vi "Host.vi"() -> ()   [LabVIEW 2018]
uses:
  <instrlib>/niDCPower/nidcpower.llb/niDCPower Source Mode.ctl
  REMOTE_SEE_CONTROLLER/RemoteSeeAbleService.dll
  <instrlib>/niDCPower/nidcpower.llb/niDCPower Measurement Type.ctl
panel:
  in  "Wait ExamineSee, ms":u32=10
  in  "Wait CheckSee, ms":u32=10
  in  "TryParrySeeDone":bool
  in  "StartTryParrySee":bool
  in  "ShutdownDone":bool
  in  "StartShutdown":bool
  in  "IsParryable":bool
  in  "ExamineSeeDone":bool
  in  "StartExamineSee":bool
  in  "CheckSeeDone":bool
  in  "StartCheckSee":bool
  in  "SeeInfo":string
  in  "IsIncomplete":bool
  in  "IsSee":bool
  in  "Wait_after, ms":u32=10
  in  "Wait before, ms":u32=10
  in  "Wait on, ms":u32=500
  in  "SEL Reset, ms":u32=500
  in  "Тип файла":enum32{"Excel", "Text"}(radio)
  in  "Стоп":bool
  in  "V1.1":bool caption="Питание"
  in  "V1.0":bool caption="Питание"
  in  "V0.1":bool caption="Питание"
  in  "V0.0":bool caption="Питание"
  out "V1.0 bulb SEL":bool
  out "V0.0 bulb SEL":bool
  in  "Лог":path
  in  "SIM_SEL":bool caption="Имитатор\nтиристора"
  in  "V1.0_selcur":dbl=0.01 caption="Порог тиристора" format="%_6p"
  in  "V0.1_selcur":dbl=0.01 caption="Порог тиристора" format="%_6p"
  in  "V1.1_selcur":dbl=0.01 caption="Порог тиристора" format="%_6p"
  in  "V0.0_selcur":dbl=0.01 caption="Порог тиристора" format="%_6p"
  out "V0.0":u16 caption="Счетчик тиристора"
  out "V1.1":u16 caption="Счетчик тиристора"
  out "V0.1":u16 caption="Счетчик тиристора"
  out "V1.0":u16 caption="Счетчик тиристора"
  out "V1.1 bulb SEL":bool
  out "V0.1 bulb SEL":bool
  in  "Питание":bool caption="Общее питание"
  in  "PXI источник №2":refnum<k15>="PXI1Slot3_3" caption="1"
  in  "PXI источник №1":refnum<k15>="PXI1Slot2_2"
  out "V0.0_char":dbl(graph)=3.090307114174992e-07
  out "V1.1_char":dbl(graph)=7.013574706441118e-05
  in  "V0.0":dbl=1.8 caption="Напряжение" format="%_6p"
  out "V0.0_cur":dbl caption="Ток" format="%_6g"
  out "V1.1_cur":dbl caption="Ток" format="%_6g"
  in  "V0.0_curlim":dbl=0.015 caption="Предел тока" format="%_6p"
  in  "V1.1_curlim":dbl=0.015 caption="Предел тока" format="%_6p"
  in  "V1.1":dbl=1.8 caption="Напряжение" format="%_6p"
  out "V0.1_char":dbl(graph)=1.1897542296492405e-06
  out "V1.0_char":dbl(graph)=9.386918666795367e-05
  in  "V0.1":dbl=1.8 caption="Напряжение" format="%_6p"
  out "V0.1_cur":dbl caption="Ток" format="%_6g"
  out "V1.0_cur":dbl caption="Ток" format="%_6g"
  in  "V0.1_curlim":dbl=0.015 caption="Предел тока" format="%_6p"
  in  "V1.0_curlim":dbl=0.015 caption="Предел тока" format="%_6p"
  in  "V1.0":dbl=1.8 caption="Напряжение" format="%_6p"
  # "Канал 1"
  # "Канал 1"
  # "Канал 2"
  # "Канал 2"
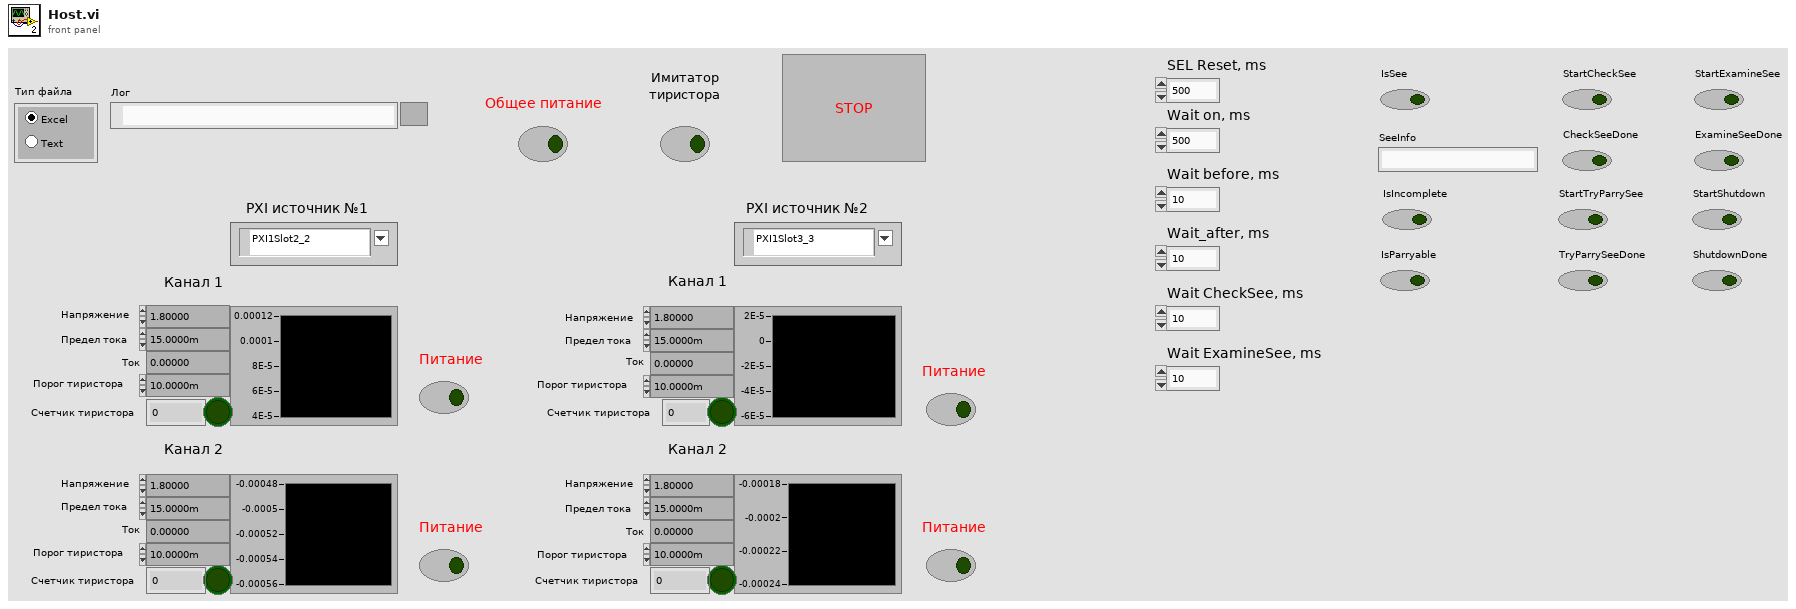
[diagram p1: front panel]
types:
  T1 = enum16{"open", "replace", "create", "open or create", "replace or create", "replace or create with confirmation"}
  T2 = typedef "niDCPower Source Mode.ctl" = i32
  T3 = cluster{"StartCheckSee":refnum<vi>, "CheckSeeDone":refnum<vi>, "IsSee":refnum<vi>, "SeeInfo":refnum<vi>, "IsIncomplete":refnum<vi>}
  T4 = cluster{"StartExamineSee":refnum<vi>, "ExamineSeeDone":refnum<vi>, "IsSee":refnum<vi>, "SeeInfo":refnum<vi>, "IsIncomplete":refnum<vi>}
  T5 = cluster{"StartShutdown":refnum<vi>, "ShutdownDone":refnum<vi>}
  T6 = cluster{"StartTryParrySee":refnum<vi>, "TryParrySeeDone":refnum<vi>}
  T7 = typedef "niDCPower Measurement Type.ctl" = i32
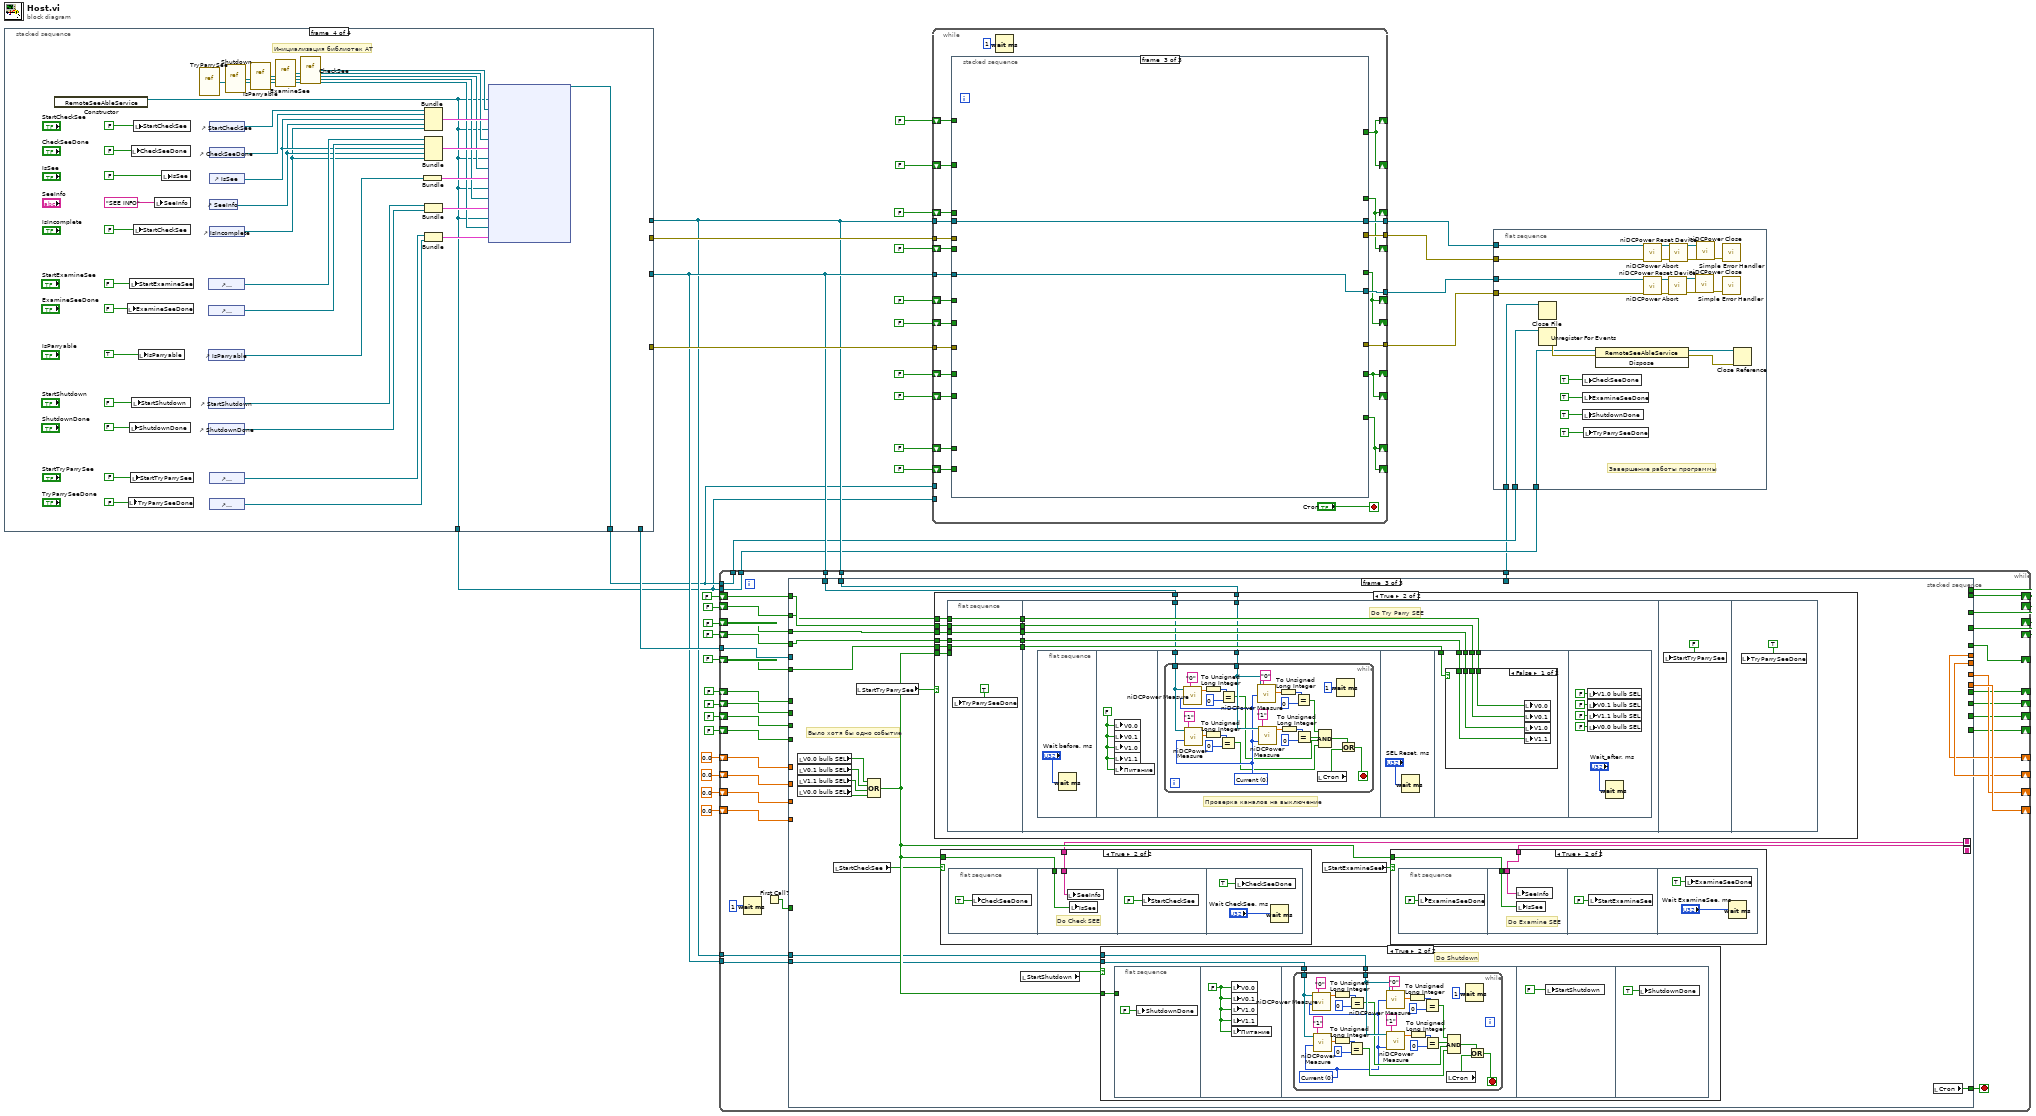
[diagram p0: block diagram]
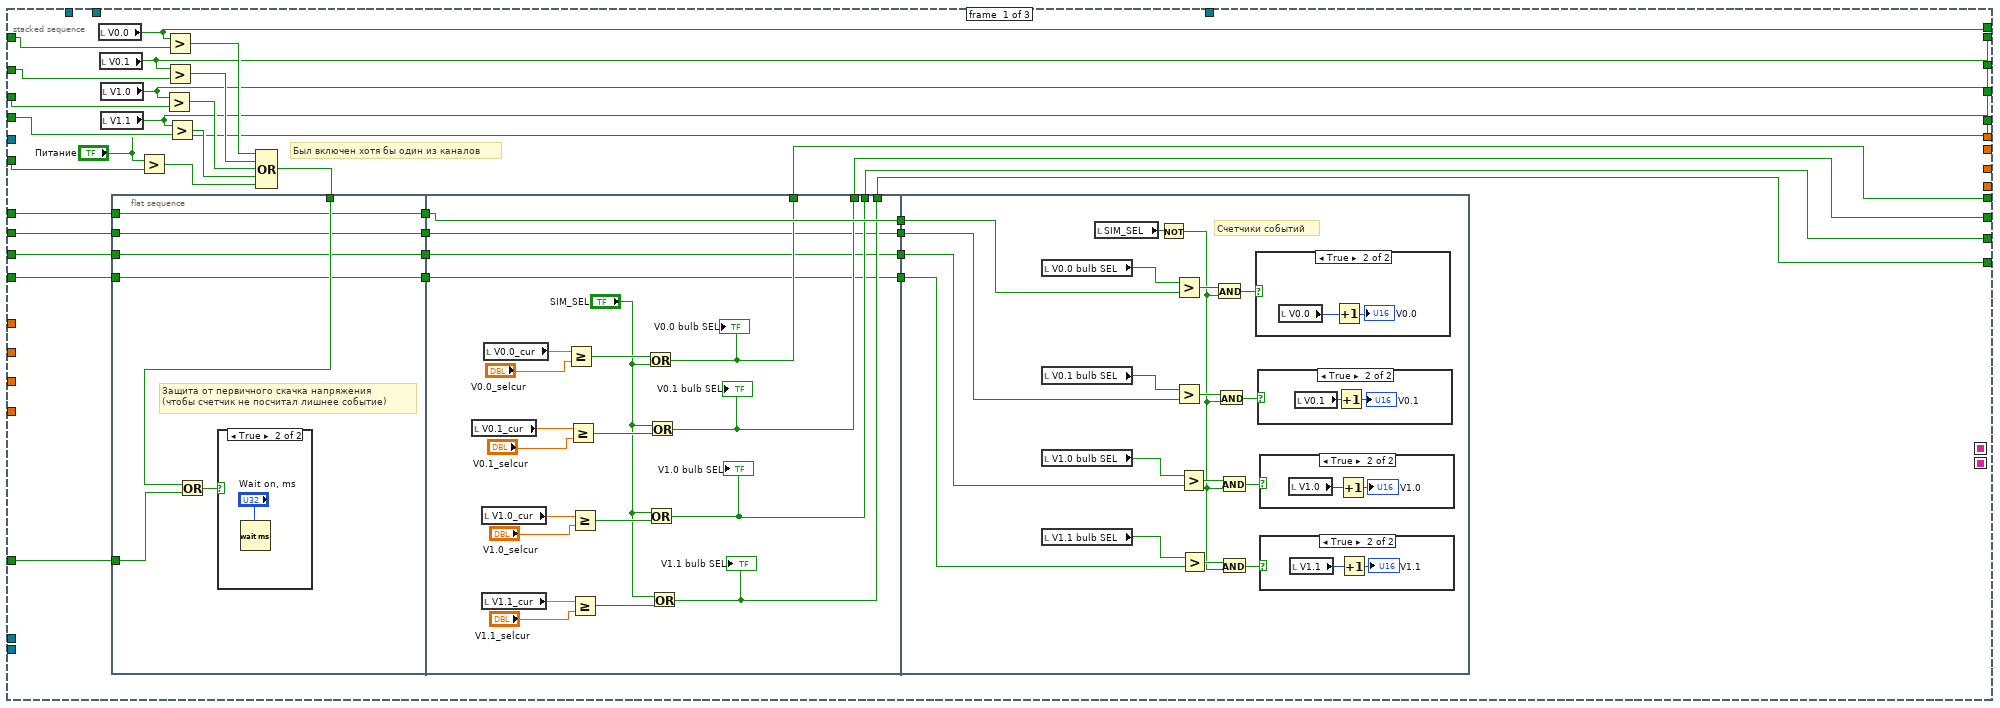
[diagram p2: hidden frame]
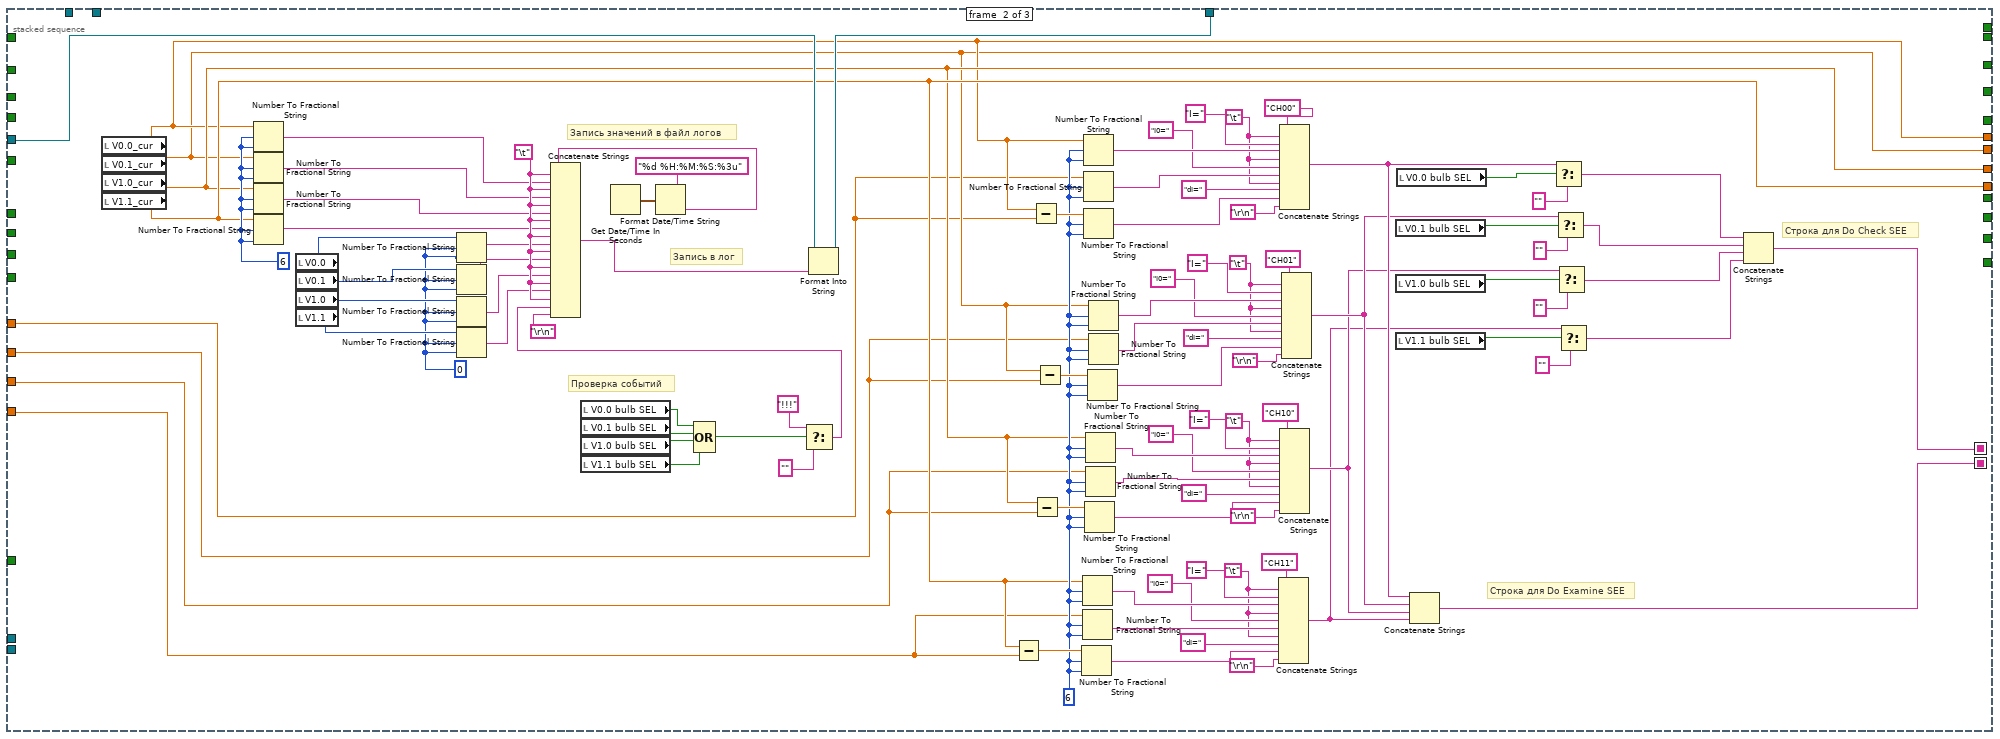
[diagram p8: hidden frame]
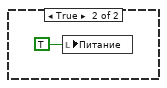
[diagram p10: hidden frame]
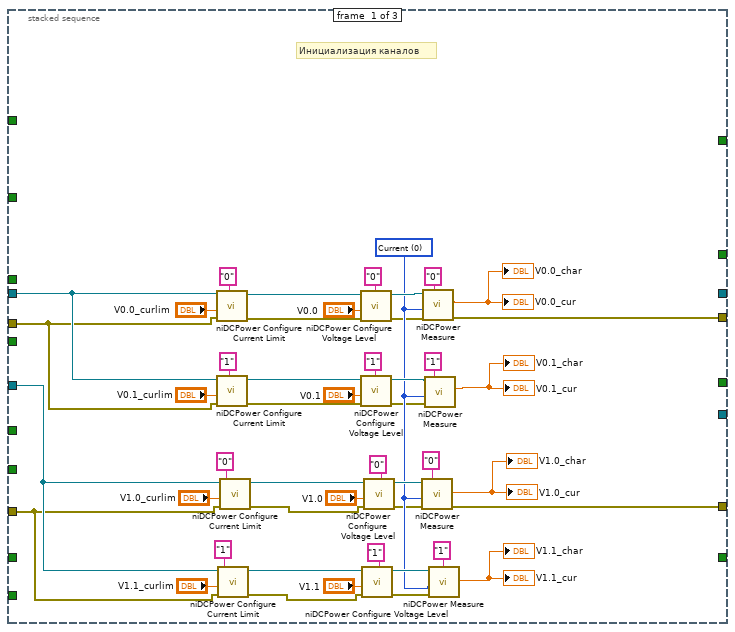
[diagram p14: hidden frame]
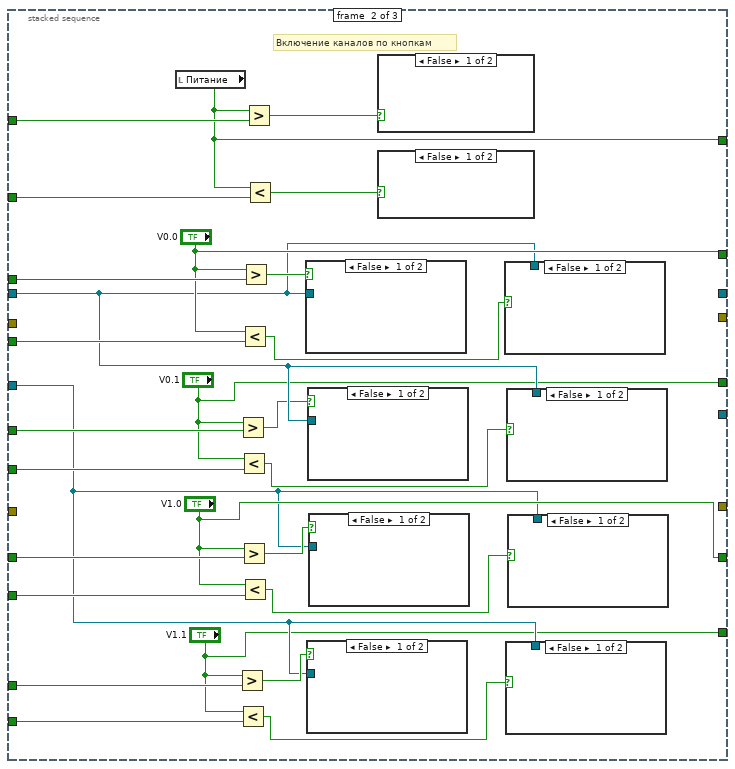
[diagram p15: hidden frame]
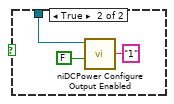
[diagram p16: hidden frame]
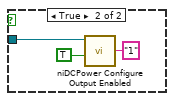
[diagram p17: hidden frame]
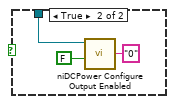
[diagram p18: hidden frame]
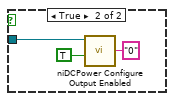
[diagram p19: hidden frame]
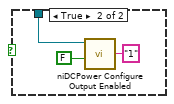
[diagram p20: hidden frame]
diagram:
  n1 = stacked-sequence {
    tunnel: [_ _ w85 _] -> w22
    tunnel: [_ _ w81 _] -> w23
    tunnel: [_ w44 _ _] -> w37
    tunnel: [_ _ w79 _] -> w29
    tunnel: [_ _ w78 _] -> w28
    tunnel: [_ _ _ w101] -> w10
    tunnel: [_ _ _ w102] -> w9
    frame #0 {
      w39 = u16 0
      w38 = FALSE
      # "Начальные значения переменных"
      n2 = local write "V1.0 bulb SEL"(w38) -> ()
      n3 = local write "V1.1 bulb SEL"(w38) -> ()
      n4 = local write "V0.0 bulb SEL"(w38) -> ()
      n5 = local write "V0.1 bulb SEL"(w38) -> ()
      n6 = local write "V0.1 bulb SEL"(w38) -> ()
      n7 = local write "Питание"(w38) -> ()
      n8 = local write "SIM_SEL"(w38) -> ()
      n9 = local write "Стоп"(w38) -> ()
      n10 = local write "V1.0"(w38) -> ()
      n11 = local write "V1.1"(w38) -> ()
      n12 = local write "V0.0"(w38) -> ()
      n13 = local write "V0.1"(w38) -> ()
      n14 = local write "V1.0"(w39) -> ()
      n15 = local write "V0.1"(w39) -> ()
      n16 = local write "V1.1"(w39) -> ()
      n17 = local write "V0.0"(w39) -> ()
    }
    frame #1 {
      w50 = "\t"
      # "Инициализация файла логов"
      n18 = call "Begin.vi"() -> ("Образец № 2"=w46:string)  [unwired: 9 in]
      n19 = Build Path(base path="Лог", name or relative path=w46) -> (appended path=w66:path)
      n20 = Get Date/Time In Seconds() -> (seconds since 1Jan1904=w63:timestamp)
      n21 = call <vilib>:"Check if File or Folder Exists.vi"("path"=w66) -> ("file or folder exists?"=w65:bool, "dup path"=w64:path)  [unwired: 8 in, 1 out]
      n22 = Format Date/Time String(time format string (%c)="%d %H.%M.%S", seconds (now)=w63) -> (date/time string=w62:string)  [unwired: 1 in]
      n23 = case shown="True" w65 {
        tunnel: w64 -> [w72 w73]
        tunnel: [w71 w73] -> w41
        frame False {
          n24 = Create Folder(path (use dialog)=w72) -> (created path=w71:path)  [unwired: 2 in, 2 out]
        }
        frame True {
        }
      }
      n25 = case shown="\"Text\"" "Тип файла" {
        tunnel: [".xls" ("string") ".txt" ("string")] -> w61
        tunnel: w41 -> [w67 w69]
        tunnel: [w67 w69] -> w40
        frame "Excel", Default {
        }
        frame "Text" {
        }
      }
      n26 = Concatenate Strings(w62, w61) -> (w59:string)
      n27 = Build Path(base path=w40, name or relative path=w59) -> (appended path=w56:path)
      n28 = Open/Create/Replace File(file path (use dialog)=w56, operation (0:open)=T1."open or create", access (0:read/write)=enum16{"read/write", "read-only", "write-only"}."read/write") -> (refnum out=w48:refnum<file>)  [unwired: 3 in, 2 out]
      n29 = Set File Position(refnum=w48, from (0:start)=enum16{"start", "end", "current"}."end") -> (refnum out=w45:refnum<file>)  [unwired: 2 in, 1 out]
      n30 = Format Into String(initial string=w45, "Time" ("string"), w50, " V 0.0" ("string"), w50, "V 0.1" ("string"), w50, "V 1.0" ("string"), w50, "V 1.1" ("string"), w50, "\r\n") -> (resulting string=w44:refnum<file>)  [unwired: 2 in, 1 out]
    }
    frame #2 {
      w86 = T2 1020 items=["Single Point"=1020, "Sequence"=1021] ("source mode")
      w92 = T2 1020 items=["Single Point"=1020, "Sequence"=1021] ("source mode")
      # "Инициализация источников"
      n31 = call <instrlib>:"niDCPower Initialize With Channels.vi"("channels"="0,1", "resource name"="PXI источник №1") -> ("error out"=w88:errorcluster, "instrument handle out"=w91:refnum<k15>)  [unwired: 8 in]
      n32 = call <instrlib>:"niDCPower Initialize With Channels.vi"("channels"="0,1", "resource name"="PXI источник №2") -> ("error out"=w93:errorcluster, "instrument handle out"=w95:refnum<k15>)  [unwired: 8 in]
      n33 = call <instrlib>:"niDCPower Configure Source Mode.vi"("error in (no error)"=w93, "source mode"=w92, "instrument handle"=w95) -> ("error out"=w87:errorcluster, "instrument handle out"=w94:refnum<k15>)  [unwired: 7 in]
      n34 = call <instrlib>:"niDCPower Configure Source Mode.vi"("error in (no error)"=w88, "source mode"=w86, "instrument handle"=w91) -> ("error out"=w89:errorcluster, "instrument handle out"=w90:refnum<k15>)  [unwired: 7 in]
      n35 = call <instrlib>:"niDCPower Configure Voltage Level.vi"("error in (no error)"=w87, "voltage level"=0.0, "channel name"="0,1", "instrument handle"=w94) -> ("error out"=w83:errorcluster, "instrument handle out"=w82:refnum<k15>)  [unwired: 6 in]
      n36 = call <instrlib>:"niDCPower Configure Voltage Level.vi"("error in (no error)"=w89, "voltage level"=0.0, "channel name"="0,1", "instrument handle"=w90) -> ("error out"=w80:errorcluster, "instrument handle out"=w84:refnum<k15>)  [unwired: 6 in]
      n37 = call <instrlib>:"niDCPower Initiate.vi"("error in (no error)"=w80, "instrument handle"=w84) -> ("error out"=w79:errorcluster, "instrument handle out"=w85:refnum<k15>)  [unwired: 2 in, 6 out]
      n38 = call <instrlib>:"niDCPower Initiate.vi"("error in (no error)"=w83, "instrument handle"=w82) -> ("error out"=w78:errorcluster, "instrument handle out"=w81:refnum<k15>)  [unwired: 2 in, 6 out]
    }
    frame #3 {
      # "Инициализация библиотек АТ"
      n39 = constructor class="RemoteSeeAbleService"() -> (reference out=w102:refnum<k24>)  [unwired: 3 in, 2 out]
      n40 = local write "ExamineSeeDone"(FALSE ("StartCheckSee")) -> ()
      n41 = local write "TryParrySeeDone"(FALSE ("StartCheckSee")) -> ()
      n42 = local write "StartExamineSee"(FALSE ("StartCheckSee")) -> ()
      n43 = local write "ShutdownDone"(FALSE ("StartCheckSee")) -> ()
      n44 = local write "StartTryParrySee"(FALSE ("StartCheckSee")) -> ()
      n45 = local write "CheckSeeDone"(FALSE ("StartCheckSee")) -> ()
      n46 = local write "StartShutdown"(FALSE ("StartCheckSee")) -> ()
      n47 = local write "StartCheckSee"(FALSE ("StartCheckSee")) -> ()
      n48 = local write "StartCheckSee"(FALSE ("StartCheckSee")) -> ()
      n49 = local write "IsParryable"(TRUE ("StartCheckSee")) -> ()
      n50 = local write "SeeInfo"("SEE INFO" ("SeeInfo")) -> ()
      n51 = local write "IsSee"(FALSE ("StartCheckSee")) -> ()
      n52 = vi-ref "TryParrySee.vi"() -> ("vi reference"=w103:refnum<vi>)
      n53 = control-ref of="StartExamineSee"() -> (w125:refnum<vi>)
      n54 = control-ref of="ExamineSeeDone"() -> (w124:refnum<vi>)
      n55 = control-ref of="IsParryable"() -> (w118:refnum<vi>)
      n56 = control-ref of="StartShutdown"() -> (w114:refnum<vi>)
      n57 = control-ref of="ShutdownDone"() -> (w113:refnum<vi>)
      n58 = control-ref of="StartCheckSee"() -> (w100:refnum<vi>)
      n59 = control-ref of="CheckSeeDone"() -> (w134:refnum<vi>)
      n60 = control-ref of="IsSee"() -> (w123:refnum<vi>)
      n61 = control-ref of="SeeInfo"() -> (w122:refnum<vi>)
      n62 = control-ref of="IsIncomplete"() -> (w121:refnum<vi>)
      n63 = control-ref of="StartTryParrySee"() -> (w109:refnum<vi>)
      n64 = control-ref of="TryParrySeeDone"() -> (w108:refnum<vi>)
      n65 = vi-ref "Shutdown.vi"() -> ("vi reference"=w104:refnum<vi>)
      n66 = vi-ref "IsParryable.vi"() -> ("vi reference"=w105:refnum<vi>)
      n67 = vi-ref "ExamineSee.vi"() -> ("vi reference"=w106:refnum<vi>)
      n68 = vi-ref "CheckSee.vi"() -> ("vi reference"=w133:refnum<vi>)
      n69 = Bundle("IsParryable"=w118) -> (w117:cluster{"IsParryable":refnum<vi>})  [unwired: 1 in]
      n70 = Bundle("StartCheckSee"=w100, "CheckSeeDone"=w134, "IsSee"=w123, "SeeInfo"=w122, "IsIncomplete"=w121) -> (w135:T3)  [unwired: 1 in]
      n71 = Bundle("StartExamineSee"=w125, "ExamineSeeDone"=w124, "IsSee"=w123, "SeeInfo"=w122, "IsIncomplete"=w121) -> (w120:T4)  [unwired: 1 in]
      n72 = Bundle("StartShutdown"=w114, "ShutdownDone"=w113) -> (w112:T5)  [unwired: 1 in]
      n73 = Bundle("StartTryParrySee"=w109, "TryParrySeeDone"=w108) -> (w107:T6)  [unwired: 1 in]
      n74 = node(w102, w133, w135, w102, w106, w120, w102, w105, w117, w102, w104, w112, w102, w103, w107) -> (w101:refnum<k27>)  [unwired: 2 in, 1 out]
    }
  }
  n75 = while {
    shift-right: [w145] -> _
    shift-left: FALSE ("V0.1") -> [w172]
    tunnel: w37 -> [w170]
    tunnel: w23 -> [w152]
    tunnel: w22 -> [w153]
    shift-right: [w163] -> _
    shift-left: FALSE ("V0.1") -> [w169]
    shift-right: [w164] -> _
    shift-left: FALSE ("V0.1") -> [w168]
    shift-right: [w165] -> _
    shift-left: FALSE ("V0.1") -> [w167]
    shift-right: [w162] -> _
    shift-left: FALSE ("V0.1") -> [w166]
    tunnel: w10 -> [w148]
    tunnel: w9 -> [w147]
    shift-right: [w159] -> _
    shift-left: 0.0 ("V0.1_cur") -> [w156]
    shift-right: [w160] -> _
    shift-left: 0.0 ("V1.0_cur") -> [w155]
    shift-right: [w161] -> _
    shift-left: 0.0 ("V1.1_cur") -> [w154]
    shift-right: [w158] -> _
    shift-left: 0.0 ("V0.0_cur") -> [w157]
    tunnel: w23 -> [w151]
    tunnel: w22 -> [w150]
    tunnel: [w148] -> w12
    tunnel: [w147] -> w11
    tunnel: [w146] -> w5
    shift-right: [w140] -> _
    shift-left: FALSE ("V0.1") -> [w144]
    shift-right: [w139] -> _
    shift-left: FALSE ("V0.1") -> [w143]
    shift-right: [w138] -> _
    shift-left: FALSE ("V0.1") -> [w142]
    shift-right: [w137] -> _
    shift-left: FALSE ("V0.1") -> [w141]
    stop <- w136 stop-if-true
    n76 = Wait (ms)(milliseconds to wait=u32 1) -> ()  [unwired: 1 out]
    n77 = First Call?() -> (First Call?: T/F=w149:bool)
    n78 = stacked-sequence {
      seq-local: [_ w275 _] -> [_ _ w371]
      seq-local: [_ w274 _] -> [_ _ w372]
      tunnel: w172 -> [w205 _ w375]
      tunnel: ["Питание" _ _] -> w145
      tunnel: w170 -> [_ w321 _]
      tunnel: [_ w345 _] -> w146
      tunnel: w169 -> [w201 _ w365]
      tunnel: w168 -> [w202 _ w364]
      tunnel: w167 -> [w203 _ w363]
      tunnel: w166 -> [w204 _ w366]
      tunnel: [w192 _ _] -> w165
      tunnel: [w191 _ _] -> w164
      tunnel: [w190 _ _] -> w163
      tunnel: [w189 _ _] -> w162
      tunnel: [_ w273 _] -> w161
      tunnel: [_ w272 _] -> w160
      tunnel: [_ w270 _] -> w159
      tunnel: [_ w271 _] -> w158
      tunnel: w157 -> [_ w269 _]
      tunnel: w156 -> [_ w268 _]
      tunnel: w155 -> [_ w267 _]
      tunnel: w154 -> [_ w266 _]
      tunnel: w153 -> [_ _ w358]
      tunnel: w152 -> [_ _ w359]
      tunnel: w151 -> [_ _ w361]
      tunnel: w150 -> [_ _ w362]
      tunnel: w149 -> [w194 _ _]
      tunnel: w144 -> [w188 _ _]
      tunnel: w143 -> [w187 _ _]
      tunnel: w142 -> [w186 _ _]
      tunnel: w141 -> [w185 _ _]
      tunnel: [w184 _ _] -> w140
      tunnel: [w183 _ _] -> w139
      tunnel: [w182 _ _] -> w138
      tunnel: [w181 _ _] -> w137
      tunnel: [_ _ w360] -> w136
      frame #0 {
        # "Был включен хотя бы один из каналов"
        n79 = local read "V0.0"() -> (w192:bool)
        n80 = local read "V0.1"() -> (w191:bool)
        n81 = local read "V1.0"() -> (w190:bool)
        n82 = local read "V1.1"() -> (w189:bool)
        n83 = flat-sequence {
          tunnel: w200 -> [w211]
          tunnel: w194 -> [w210]
          tunnel: w188 -> [w209]
          tunnel: w187 -> [w208]
          tunnel: w186 -> [w207]
          tunnel: w185 -> [w206]
          tunnel: [w209] -> w179
          tunnel: [w208] -> w178
          tunnel: [w207] -> w177
          tunnel: [w206] -> w176
          tunnel: w179 -> [w226]
          tunnel: w178 -> [w216]
          tunnel: w177 -> [w215]
          tunnel: w176 -> [w214]
          tunnel: [w224] -> w184
          tunnel: [w222] -> w183
          tunnel: [w220] -> w182
          tunnel: [w221] -> w181
          tunnel: [w226] -> w180
          tunnel: [w216] -> w175
          tunnel: [w215] -> w174
          tunnel: [w214] -> w173
          tunnel: w180 -> [w251]
          tunnel: w175 -> [w249]
          tunnel: w174 -> [w247]
          tunnel: w173 -> [w245]
          frame #0 {
            # "Защита от первичного скачка напряжения\n(чтобы счетчик не посчитал лишнее событие)"
            n84 = Or(x=w211, y=w210) -> (x .or. y?=w212:bool)
            n85 = case shown="True" w212 {
              frame False {
              }
              frame True {
                n86 = Wait (ms)(milliseconds to wait="Wait on, ms") -> ()  [unwired: 1 out]
              }
            }
          }
          frame #1 {
            n87 = local read "V0.1_cur"() -> (w227:dbl)
            n88 = local read "V1.0_cur"() -> (w233:dbl)
            n89 = local read "V1.1_cur"() -> (w228:dbl)
            n90 = local read "V0.0_cur"() -> (w231:dbl)
            n91 = Greater Or Equal?(x=w231, y="V0.0_selcur") -> (x >= y?=w225:bool)
            n92 = Greater Or Equal?(x=w227, y="V0.1_selcur") -> (x >= y?=w223:bool)
            n93 = Greater Or Equal?(x=w233, y="V1.0_selcur") -> (x >= y?=w219:bool)
            n94 = Greater Or Equal?(x=w228, y="V1.1_selcur") -> (x >= y?=w218:bool)
            n95 = Or(x=w225, y="SIM_SEL") -> (x .or. y?=w224:bool)
            "V0.0 bulb SEL" <- w224
            n96 = Or(x="SIM_SEL", y=w219) -> (x .or. y?=w220:bool)
            "V1.0 bulb SEL" <- w220
            n97 = Or(x="SIM_SEL", y=w223) -> (x .or. y?=w222:bool)
            "V0.1 bulb SEL" <- w222
            n98 = Or(x="SIM_SEL", y=w218) -> (x .or. y?=w221:bool)
            "V1.1 bulb SEL" <- w221
          }
          frame #2 {
            # "Счетчики событий"
            n99 = local read "V0.0 bulb SEL"() -> (w252:bool)
            n100 = local read "V0.1 bulb SEL"() -> (w250:bool)
            n101 = local read "V1.0 bulb SEL"() -> (w248:bool)
            n102 = local read "V1.1 bulb SEL"() -> (w246:bool)
            n103 = local read "SIM_SEL"() -> (w236:bool)
            n104 = Not(x=w236) -> (.not. x?=w235:bool)
            n105 = Greater?(x=w252, y=w251) -> (0:w244:bool)
            n106 = Greater?(x=w250, y=w249) -> (0:w237:bool)
            n107 = Greater?(x=w248, y=w247) -> (0:w238:bool)
            n108 = Greater?(x=w246, y=w245) -> (0:w239:bool)
            n109 = And(x=w244, y=w235) -> (x .and. y?=w243:bool)
            n110 = And(x=w237, y=w235) -> (x .and. y?=w242:bool)
            n111 = And(x=w238, y=w235) -> (x .and. y?=w241:bool)
            n112 = And(x=w239, y=w235) -> (x .and. y?=w240:bool)
            n113 = case shown="True" w243 {
              frame False {
              }
              frame True {
                n114 = local read "V0.0"() -> (w256:u16)
                n115 = Increment(x=w256) -> (x+1=→"V0.0":u16)
              }
            }
            n116 = case shown="True" w242 {
              frame False {
              }
              frame True {
                n117 = local read "V0.1"() -> (w258:u16)
                n118 = Increment(x=w258) -> (x+1=→"V0.1":u16)
              }
            }
            n119 = case shown="True" w241 {
              frame False {
              }
              frame True {
                n120 = local read "V1.0"() -> (w253:u16)
                n121 = Increment(x=w253) -> (x+1=→"V1.0":u16)
              }
            }
            n122 = case shown="True" w240 {
              frame False {
              }
              frame True {
                n123 = local read "V1.1"() -> (w260:u16)
                n124 = Increment(x=w260) -> (x+1=→"V1.1":u16)
              }
            }
          }
        }
        n125 = Greater?(x="Питание", y=w205) -> (0:w199:bool)
        n126 = Greater?(x=w190, y=w201) -> (0:w197:bool)
        n127 = Greater?(x=w192, y=w203) -> (0:w195:bool)
        n128 = Greater?(x=w191, y=w202) -> (0:w196:bool)
        n129 = Greater?(x=w189, y=w204) -> (0:w198:bool)
        n130 = Compound Arithmetic op=OR(w195, w196, w197, w198, w199) -> (w200:bool)
      }
      frame #1 {
        w277 = "\t"
        w281 = "\t"
        w285 = "\t"
        w290 = "\t"
        w328 = 6
        w276 = 0
        w353 = 6
        w354 = "\t"
        # "Проверка событий"
        # "Запись значений в файл логов"
        # "Запись в лог"
        # "Строка для Do Check SEE"
        # "Строка для Do Examine SEE"
        n131 = local read "V0.0_cur"() -> (w271:dbl)
        n132 = local read "V0.1_cur"() -> (w270:dbl)
        n133 = local read "V1.0_cur"() -> (w272:dbl)
        n134 = local read "V1.1_cur"() -> (w273:dbl)
        n135 = Number To Fractional String(number=w271, width (-)=w353, precision (6)=w353) -> (F-format string=w338:string)  [unwired: 1 in]
        n136 = Number To Fractional String(number=w270, width (-)=w353, precision (6)=w353) -> (F-format string=w337:string)  [unwired: 1 in]
        n137 = Number To Fractional String(number=w272, width (-)=w353, precision (6)=w353) -> (F-format string=w336:string)  [unwired: 1 in]
        n138 = Number To Fractional String(number=w273, width (-)=w353, precision (6)=w353) -> (F-format string=w334:string)  [unwired: 1 in]
        n139 = local read "V0.0"() -> (w344:u16)
        n140 = local read "V0.1"() -> (w343:u16)
        n141 = local read "V1.0"() -> (w342:u16)
        n142 = local read "V1.1"() -> (w341:u16)
        n143 = Number To Fractional String(number=w344, width (-)=w276, precision (6)=w276) -> (F-format string=w351:string)  [unwired: 1 in]
        n144 = Number To Fractional String(number=w343, width (-)=w276, precision (6)=w276) -> (F-format string=w350:string)  [unwired: 1 in]
        n145 = Number To Fractional String(number=w342, width (-)=w276, precision (6)=w276) -> (F-format string=w349:string)  [unwired: 1 in]
        n146 = Number To Fractional String(number=w341, width (-)=w276, precision (6)=w276) -> (F-format string=w348:string)  [unwired: 1 in]
        n147 = local read "V0.0 bulb SEL"() -> (w262:bool)
        n148 = local read "V0.1 bulb SEL"() -> (w308:bool)
        n149 = local read "V1.0 bulb SEL"() -> (w307:bool)
        n150 = local read "V1.1 bulb SEL"() -> (w306:bool)
        n151 = Get Date/Time In Seconds() -> (seconds since 1Jan1904=w356:timestamp)
        n152 = Format Date/Time String(time format string (%c)="%d %H:%M:%S:%3u", seconds (now)=w356) -> (date/time string=w339:string)  [unwired: 1 in]
        n153 = Compound Arithmetic op=OR(w262, w308, w307, w306) -> (w297:bool)
        n154 = Select(t="!!!", s=w297, f="") -> (s? t:f=w347:string)
        n155 = Concatenate Strings(w339, w354, w338, w354, w337, w354, w336, w354, w334, w354, w351, w354, w350, w354, w349, w354, w348, w354, w347, "\r\n") -> (w340:string)
        n156 = Format Into String(initial string=w321, w340) -> (resulting string=w345:refnum<file>)  [unwired: 2 in, 1 out]
        n157 = Subtract(x=w273, y=w266) -> (x-y=w329:dbl)
        n158 = Subtract(x=w271, y=w269) -> (x-y=w335:dbl)
        n159 = Subtract(x=w272, y=w267) -> (x-y=w330:dbl)
        n160 = Subtract(x=w270, y=w268) -> (x-y=w331:dbl)
        n161 = Number To Fractional String(number=w329, width (-)=w328, precision (6)=w328) -> (F-format string=w279:string)  [unwired: 1 in]
        n162 = Number To Fractional String(number=w273, width (-)=w328, precision (6)=w328) -> (F-format string=w326:string)  [unwired: 1 in]
        n163 = Number To Fractional String(number=w266, width (-)=w328, precision (6)=w328) -> (F-format string=w327:string)  [unwired: 1 in]
        n164 = Number To Fractional String(number=w271, width (-)=w328, precision (6)=w328) -> (F-format string=w333:string)  [unwired: 1 in]
        n165 = Number To Fractional String(number=w269, width (-)=w328, precision (6)=w328) -> (F-format string=w332:string)  [unwired: 1 in]
        n166 = Number To Fractional String(number=w335, width (-)=w328, precision (6)=w328) -> (F-format string=w292:string)  [unwired: 1 in]
        n167 = Number To Fractional String(number=w330, width (-)=w328, precision (6)=w328) -> (F-format string=w283:string)  [unwired: 1 in]
        n168 = Number To Fractional String(number=w272, width (-)=w328, precision (6)=w328) -> (F-format string=w324:string)  [unwired: 1 in]
        n169 = Number To Fractional String(number=w267, width (-)=w328, precision (6)=w328) -> (F-format string=w325:string)  [unwired: 1 in]
        n170 = Number To Fractional String(number=w331, width (-)=w328, precision (6)=w328) -> (F-format string=w287:string)  [unwired: 1 in]
        n171 = Number To Fractional String(number=w270, width (-)=w328, precision (6)=w328) -> (F-format string=w322:string)  [unwired: 1 in]
        n172 = Number To Fractional String(number=w268, width (-)=w328, precision (6)=w328) -> (F-format string=w323:string)  [unwired: 1 in]
        n173 = Concatenate Strings("CH11" ("string"), w277, "I=", w326, w277, "I0=", w327, w277, "dI=", w279, "\r\n") -> (w302:string)
        n174 = Concatenate Strings("CH00" ("string"), w290, "I=", w333, w290, "I0=", w332, w290, "dI=", w292, "\r\n") -> (w305:string)
        n175 = Concatenate Strings("CH10" ("string"), w281, "I=", w324, w281, "I0=", w325, w281, "dI=", w283, "\r\n") -> (w303:string)
        n176 = Concatenate Strings("CH01" ("string"), w285, "I=", w322, w285, "I0=", w323, w285, "dI=", w287, "\r\n") -> (w304:string)
        n177 = local read "V0.1 bulb SEL"() -> (w265:bool)
        n178 = local read "V1.0 bulb SEL"() -> (w264:bool)
        n179 = local read "V1.1 bulb SEL"() -> (w263:bool)
        n180 = local read "V0.0 bulb SEL"() -> (w261:bool)
        n181 = Concatenate Strings(w305, w304, w303, w302) -> (w275:string)
        n182 = Select(t=w305, s=w261, f="") -> (s? t:f=w296:string)
        n183 = Select(t=w304, s=w265, f="") -> (s? t:f=w295:string)
        n184 = Select(t=w303, s=w264, f="") -> (s? t:f=w294:string)
        n185 = Select(t=w302, s=w263, f="") -> (s? t:f=w293:string)
        n186 = Concatenate Strings(w296, w295, w294, w293) -> (w274:string)
      }
      frame #2 {
        # "Было хотя бы одно событие"
        n187 = local read "V0.0 bulb SEL"() -> (w370:bool)
        n188 = local read "V0.1 bulb SEL"() -> (w378:bool)
        n189 = local read "V1.1 bulb SEL"() -> (w376:bool)
        n190 = local read "V0.0 bulb SEL"() -> (w377:bool)
        n191 = local read "StartCheckSee"() -> (w369:bool)
        n192 = local read "StartTryParrySee"() -> (w367:bool)
        n193 = Compound Arithmetic op=OR(w370, w378, w376, w377) -> (w373:bool)
        n194 = case shown="True" w367 {
          tunnel: w373 -> [_ w391]
          tunnel: w375 -> [_ w389]
          tunnel: w366 -> [_ w387]
          tunnel: w365 -> [_ w385]
          tunnel: w364 -> [_ w383]
          tunnel: w363 -> [_ w381]
          tunnel: w362 -> [_ w380]
          tunnel: w361 -> [_ w379]
          frame False {
          }
          frame True {
            n195 = flat-sequence {
              tunnel: w391 -> [_]
              tunnel: [w396] -> w390
              tunnel: w389 -> [w396]
              tunnel: [w395] -> w388
              tunnel: w387 -> [w395]
              tunnel: [w394] -> w386
              tunnel: w385 -> [w394]
              tunnel: [w393] -> w384
              tunnel: w383 -> [w393]
              tunnel: [w392] -> w382
              tunnel: w381 -> [w392]
              tunnel: w390 -> [w400]
              tunnel: w388 -> [w401]
              tunnel: w386 -> [w402]
              tunnel: w384 -> [w403]
              tunnel: w382 -> [w404]
              tunnel: w380 -> [w399]
              tunnel: w379 -> [w398]
              frame #0 {
                n196 = local write "TryParrySeeDone"(TRUE ("StartCheckSee")) -> ()
              }
              frame #1 {
                # "Do Try Parry SEE"
                n197 = flat-sequence {
                  tunnel: w399 -> [w408]
                  tunnel: w398 -> [w407]
                  tunnel: w404 -> [w441]
                  tunnel: w403 -> [w440]
                  tunnel: w402 -> [w439]
                  tunnel: w401 -> [w438]
                  tunnel: w400 -> [w437]
                  frame #0 {
                    n198 = Wait (ms)(milliseconds to wait="Wait before, ms") -> ()  [unwired: 1 out]
                  }
                  frame #1 {
                    w406 = FALSE ("Линейки")
                    n199 = local write "V0.0"(w406) -> ()
                    n200 = local write "V0.1"(w406) -> ()
                    n201 = local write "V1.0"(w406) -> ()
                    n202 = local write "V1.1"(w406) -> ()
                    n203 = local write "Питание"(w406) -> ()
                  }
                  frame #2 {
                    # "Проверка каналов на выключение"
                    n204 = while {
                      tunnel: w408 -> [w432]
                      tunnel: w407 -> [w429]
                      stop <- w435 stop-if-true
                      w426 = T7 0 items=["Current", "Voltage"] ("measurement type")
                      n205 = call <instrlib>:"niDCPower Measure.vi"("measurement type"=w426, "channel name"="0", "instrument handle"=w429) -> ("measurement"=w418:dbl)  [unwired: 6 in, 2 out]
                      n206 = call <instrlib>:"niDCPower Measure.vi"("measurement type"=w426, "channel name"="1", "instrument handle"=w429) -> ("measurement"=w414:dbl)  [unwired: 6 in, 2 out]
                      n207 = To Unsigned Long Integer(number=w414) -> (unsigned 32bit integer=w415:u32)
                      n208 = To Unsigned Long Integer(number=w418) -> (unsigned 32bit integer=w420:u32)
                      n209 = Equal?(x=w415, y=u32 0) -> (x = y?=w413:bool)
                      n210 = Equal?(x=w420, y=u32 0) -> (x = y?=w417:bool)
                      n211 = call <instrlib>:"niDCPower Measure.vi"("measurement type"=w426, "channel name"="0", "instrument handle"=w432) -> ("measurement"=w423:dbl)  [unwired: 6 in, 2 out]
                      n212 = call <instrlib>:"niDCPower Measure.vi"("measurement type"=w426, "channel name"="1", "instrument handle"=w432) -> ("measurement"=w409:dbl)  [unwired: 6 in, 2 out]
                      n213 = To Unsigned Long Integer(number=w423) -> (unsigned 32bit integer=w422:u32)
                      n214 = To Unsigned Long Integer(number=w409) -> (unsigned 32bit integer=w412:u32)
                      n215 = Equal?(x=w422, y=u32 0) -> (x = y?=w421:bool)
                      n216 = Equal?(x=w412, y=u32 0) -> (x = y?=w410:bool)
                      n217 = local read "Стоп"() -> (w428:bool)
                      n218 = Compound Arithmetic op=AND(w421, w410, w417, w413) -> (w427:bool)
                      n219 = Wait (ms)(milliseconds to wait=u32 1) -> ()  [unwired: 1 out]
                      n220 = Or(x=w427, y=w428) -> (x .or. y?=w435:bool)
                    }
                  }
                  frame #3 {
                    n221 = Wait (ms)(milliseconds to wait="SEL Reset, ms") -> ()  [unwired: 1 out]
                  }
                  frame #4 {
                    n222 = case shown="False" w437 {
                      tunnel: w441 -> [w445 _]
                      tunnel: w440 -> [w444 _]
                      tunnel: w439 -> [w443 _]
                      tunnel: w438 -> [w442 _]
                      frame False {
                        n223 = local write "V0.0"(w445) -> ()
                        n224 = local write "V0.1"(w444) -> ()
                        n225 = local write "V1.0"(w443) -> ()
                        n226 = local write "V1.1"(w442) -> ()
                      }
                      frame True {
                        n227 = local write "Питание"(TRUE ("Линейки")) -> ()
                      }
                    }
                  }
                  frame #5 {
                    n228 = local write "V1.0 bulb SEL"(FALSE ("V1.0 bulb SEL")) -> ()
                    n229 = local write "V0.1 bulb SEL"(FALSE ("V0.1 bulb SEL")) -> ()
                    n230 = local write "V1.1 bulb SEL"(FALSE ("V1.1 bulb SEL")) -> ()
                    n231 = local write "V0.0 bulb SEL"(FALSE ("V0.0 bulb SEL")) -> ()
                    n232 = Wait (ms)(milliseconds to wait="Wait_after, ms") -> ()  [unwired: 1 out]
                  }
                }
              }
              frame #2 {
                n233 = local write "StartTryParrySee"(FALSE ("StartCheckSee")) -> ()
              }
              frame #3 {
                n234 = local write "TryParrySeeDone"(TRUE ("StartCheckSee")) -> ()
              }
            }
          }
        }
        n235 = case shown="True" w369 {
          tunnel: w373 -> [_ w498]
          tunnel: w372 -> [_ w499]
          frame False {
          }
          frame True {
            n236 = flat-sequence {
              tunnel: w499 -> [w502]
              tunnel: w498 -> [w501]
              frame #0 {
                n237 = local write "CheckSeeDone"(TRUE ("StartCheckSee")) -> ()
              }
              frame #1 {
                # "Do Check SEE"
                n238 = local write "SeeInfo"(w502) -> ()
                n239 = local write "IsSee"(w501) -> ()
              }
              frame #2 {
                n240 = local write "StartCheckSee"(FALSE ("StartCheckSee")) -> ()
              }
              frame #3 {
                n241 = local write "CheckSeeDone"(TRUE ("StartCheckSee")) -> ()
                n242 = Wait (ms)(milliseconds to wait="Wait CheckSee, ms") -> ()  [unwired: 1 out]
              }
            }
          }
        }
        n243 = local read "StartShutdown"() -> (w374:bool)
        n244 = case shown="True" w374 {
          tunnel: w359 -> [_ w456]
          tunnel: w373 -> [_ w455]
          tunnel: w358 -> [_ w454]
          frame False {
          }
          frame True {
            # "Do Shutdown"
            n245 = flat-sequence {
              tunnel: w455 -> [_]
              tunnel: w454 -> [w460]
              tunnel: w456 -> [w459]
              frame #0 {
                n246 = local write "ShutdownDone"(FALSE ("StartCheckSee")) -> ()
              }
              frame #1 {
                w458 = FALSE ("Линейки")
                n247 = local write "V0.0"(w458) -> ()
                n248 = local write "V0.1"(w458) -> ()
                n249 = local write "V1.0"(w458) -> ()
                n250 = local write "V1.1"(w458) -> ()
                n251 = local write "Питание"(w458) -> ()
              }
              frame #2 {
                n252 = while {
                  tunnel: w460 -> [w484]
                  tunnel: w459 -> [w481]
                  stop <- w487 stop-if-true
                  w461 = T7 0 items=["Current", "Voltage"] ("measurement type")
                  n253 = call <instrlib>:"niDCPower Measure.vi"("measurement type"=w461, "channel name"="0", "instrument handle"=w481) -> ("measurement"=w471:dbl)  [unwired: 6 in, 2 out]
                  n254 = call <instrlib>:"niDCPower Measure.vi"("measurement type"=w461, "channel name"="1", "instrument handle"=w481) -> ("measurement"=w467:dbl)  [unwired: 6 in, 2 out]
                  n255 = To Unsigned Long Integer(number=w467) -> (unsigned 32bit integer=w468:u32)
                  n256 = To Unsigned Long Integer(number=w471) -> (unsigned 32bit integer=w473:u32)
                  n257 = Equal?(x=w468, y=u32 0) -> (x = y?=w466:bool)
                  n258 = Equal?(x=w473, y=u32 0) -> (x = y?=w470:bool)
                  n259 = call <instrlib>:"niDCPower Measure.vi"("measurement type"=w461, "channel name"="0", "instrument handle"=w484) -> ("measurement"=w476:dbl)  [unwired: 6 in, 2 out]
                  n260 = call <instrlib>:"niDCPower Measure.vi"("measurement type"=w461, "channel name"="1", "instrument handle"=w484) -> ("measurement"=w462:dbl)  [unwired: 6 in, 2 out]
                  n261 = To Unsigned Long Integer(number=w476) -> (unsigned 32bit integer=w475:u32)
                  n262 = To Unsigned Long Integer(number=w462) -> (unsigned 32bit integer=w465:u32)
                  n263 = Equal?(x=w475, y=u32 0) -> (x = y?=w474:bool)
                  n264 = Equal?(x=w465, y=u32 0) -> (x = y?=w463:bool)
                  n265 = local read "Стоп"() -> (w480:bool)
                  n266 = Compound Arithmetic op=AND(w474, w463, w470, w466) -> (w479:bool)
                  n267 = Wait (ms)(milliseconds to wait=u32 1) -> ()  [unwired: 1 out]
                  n268 = Or(x=w479, y=w480) -> (x .or. y?=w487:bool)
                }
              }
              frame #3 {
                n269 = local write "StartShutdown"(FALSE ("StartCheckSee")) -> ()
              }
              frame #4 {
                n270 = local write "ShutdownDone"(TRUE ("StartCheckSee")) -> ()
              }
            }
          }
        }
        n271 = local read "StartExamineSee"() -> (w368:bool)
        n272 = case shown="True" w368 {
          tunnel: w371 -> [_ w491]
          tunnel: w373 -> [_ w490]
          frame False {
          }
          frame True {
            n273 = flat-sequence {
              tunnel: w491 -> [w494]
              tunnel: w490 -> [w493]
              frame #0 {
                n274 = local write "ExamineSeeDone"(FALSE ("StartCheckSee")) -> ()
              }
              frame #1 {
                # "Do Examine SEE"
                n275 = local write "SeeInfo"(w494) -> ()
                n276 = local write "IsSee"(w493) -> ()
              }
              frame #2 {
                n277 = local write "StartExamineSee"(FALSE ("StartCheckSee")) -> ()
              }
              frame #3 {
                n278 = local write "ExamineSeeDone"(TRUE ("StartCheckSee")) -> ()
                n279 = Wait (ms)(milliseconds to wait="Wait ExamineSee, ms") -> ()  [unwired: 1 out]
              }
            }
          }
        }
        n280 = local read "Стоп"() -> (w360:bool)
      }
    }
  }
  n281 = while {
    tunnel: w22 -> [w530]
    tunnel: w23 -> [w529]
    tunnel: [w528] -> w6
    tunnel: [w527] -> w8
    shift-right: [w524] -> _
    shift-left: FALSE -> [w526]
    shift-right: [w524] -> _
    shift-left: FALSE -> [w525]
    tunnel: w29 -> [w523]
    tunnel: [w522] -> w7
    tunnel: w28 -> [w521]
    tunnel: [w520] -> w13
    shift-right: [w515] -> _
    shift-left: FALSE -> [w518]
    shift-right: [w515] -> _
    shift-left: FALSE -> [w516]
    shift-right: [w509] -> _
    shift-left: FALSE -> [w514]
    shift-right: [w509] -> _
    shift-left: FALSE -> [w513]
    shift-right: [w510] -> _
    shift-left: FALSE -> [w512]
    shift-right: [w510] -> _
    shift-left: FALSE -> [w511]
    shift-right: [w506] -> _
    shift-left: FALSE -> [w508]
    shift-right: [w506] -> _
    shift-left: FALSE -> [w507]
    tunnel: w10 -> [_]
    tunnel: w9 -> [_]
    stop <- "Стоп" stop-if-true
    n282 = stacked-sequence {
      tunnel: w530 -> [w557 w594 w632]
      tunnel: w529 -> [w556 w580 w631]
      tunnel: [_ _ w632] -> w528
      tunnel: [_ _ w631] -> w527
      tunnel: w526 -> [_ w602 _]
      tunnel: w525 -> [_ w601 _]
      tunnel: [_ w600 _] -> w524
      tunnel: w523 -> [w536 _ _]
      tunnel: [w540 _ _] -> w522
      tunnel: w521 -> [w532 _ _]
      tunnel: [w537 _ _] -> w520
      tunnel: w518 -> [_ w599 _]
      tunnel: [_ "V0.0" _] -> w515
      tunnel: w516 -> [_ w597 _]
      tunnel: w514 -> [_ w593 _]
      tunnel: [_ "V0.1" _] -> w509
      tunnel: w513 -> [_ w590 _]
      tunnel: w512 -> [_ w587 _]
      tunnel: [_ "V1.0" _] -> w510
      tunnel: w511 -> [_ w585 _]
      tunnel: w508 -> [_ w584 _]
      tunnel: w507 -> [_ w583 _]
      tunnel: [_ "V1.1" _] -> w506
      frame #0 {
        w543 = T7 0 items=["Current", "Voltage"] ("measurement type")
        # "Инициализация каналов"
        n283 = call <instrlib>:"niDCPower Configure Current Limit.vi"("error in (no error)"=w536, "current limit"="V0.0_curlim", "channel name"="0", "instrument handle"=w557) -> ("error out"=w542:errorcluster, "instrument handle out"=w561:refnum<k15>)  [unwired: 6 in]
        n284 = call <instrlib>:"niDCPower Configure Current Limit.vi"("error in (no error)"=w536, "current limit"="V0.1_curlim", "channel name"="1", "instrument handle"=w557) -> ("error out"=w535:errorcluster, "instrument handle out"=w574:refnum<k15>)  [unwired: 6 in]
        n285 = call <instrlib>:"niDCPower Configure Current Limit.vi"("error in (no error)"=w532, "current limit"="V1.1_curlim", "channel name"="1", "instrument handle"=w556) -> ("error out"=w531:errorcluster, "instrument handle out"=w562:refnum<k15>)  [unwired: 6 in]
        n286 = call <instrlib>:"niDCPower Configure Current Limit.vi"("error in (no error)"=w532, "current limit"="V1.0_curlim", "channel name"="0", "instrument handle"=w556) -> ("error out"=w539:errorcluster, "instrument handle out"=w573:refnum<k15>)  [unwired: 6 in]
        n287 = call <instrlib>:"niDCPower Configure Voltage Level.vi"("error in (no error)"=w542, "voltage level"="V0.0", "channel name"="0", "instrument handle"=w561) -> ("error out"=w541:errorcluster, "instrument handle out"=w547:refnum<k15>)  [unwired: 6 in]
        n288 = call <instrlib>:"niDCPower Configure Voltage Level.vi"("error in (no error)"=w535, "voltage level"="V0.1", "channel name"="1", "instrument handle"=w574) -> ("error out"=w534:errorcluster, "instrument handle out"=w551:refnum<k15>)  [unwired: 6 in]
        n289 = call <instrlib>:"niDCPower Configure Voltage Level.vi"("error in (no error)"=w531, "voltage level"="V1.1", "channel name"="1", "instrument handle"=w562) -> ("error out"=w533:errorcluster, "instrument handle out"=w555:refnum<k15>)  [unwired: 6 in]
        n290 = call <instrlib>:"niDCPower Configure Voltage Level.vi"("error in (no error)"=w539, "voltage level"="V1.0", "channel name"="0", "instrument handle"=w573) -> ("error out"=w538:errorcluster, "instrument handle out"=w553:refnum<k15>)  [unwired: 6 in]
        n291 = call <instrlib>:"niDCPower Measure.vi"("error in (no error)"=w538, "measurement type"=w543, "channel name"="0", "instrument handle"=w553) -> ("error out"=w537:errorcluster, "measurement"=→"V1.0_cur" →"V1.0_char":dbl)  [unwired: 5 in, 1 out]
        n292 = call <instrlib>:"niDCPower Measure.vi"("error in (no error)"=w541, "measurement type"=w543, "channel name"="0", "instrument handle"=w547) -> ("error out"=w540:errorcluster, "measurement"=→"V0.0_cur" →"V0.0_char":dbl)  [unwired: 5 in, 1 out]
        n293 = call <instrlib>:"niDCPower Measure.vi"("error in (no error)"=w534, "measurement type"=w543, "channel name"="1", "instrument handle"=w551) -> ("measurement"=→"V0.1_cur" →"V0.1_char":dbl)  [unwired: 5 in, 2 out]
        n294 = call <instrlib>:"niDCPower Measure.vi"("error in (no error)"=w533, "measurement type"=w543, "channel name"="1", "instrument handle"=w555) -> ("measurement"=→"V1.1_cur" →"V1.1_char":dbl)  [unwired: 5 in, 2 out]
      }
      frame #1 {
        # "Включение каналов по кнопкам"
        n295 = local read "Питание"() -> (w600:bool)
        n296 = Greater?(x="V1.1", y=w584) -> (0:w582:bool)
        n297 = Greater?(x="V0.1", y=w593) -> (0:w592:bool)
        n298 = Less?(x="V1.1", y=w583) -> (x < y?=w581:bool)
        n299 = Less?(x="V0.1", y=w590) -> (x < y?=w591:bool)
        n300 = Greater?(x="V1.0", y=w587) -> (0:w589:bool)
        n301 = Less?(x="V0.0", y=w597) -> (x < y?=w595:bool)
        n302 = Less?(x="V1.0", y=w585) -> (x < y?=w588:bool)
        n303 = Greater?(x="V0.0", y=w599) -> (0:w598:bool)
        n304 = Greater?(x=w600, y=w602) -> (0:w604:bool)
        n305 = Less?(x=w600, y=w601) -> (x < y?=w603:bool)
        n306 = case shown="False" w598 {
          tunnel: w594 -> [_ w626]
          frame False {
          }
          frame True {
            n307 = call <instrlib>:"niDCPower Configure Output Enabled.vi"("output enabled"=TRUE ("V0.0"), "channel name"="0", "instrument handle"=w626) -> ()  [unwired: 7 in, 2 out]
          }
        }
        n308 = case shown="False" w582 {
          tunnel: w580 -> [_ w608]
          frame False {
          }
          frame True {
            n309 = call <instrlib>:"niDCPower Configure Output Enabled.vi"("output enabled"=TRUE ("V0.0"), "channel name"="1", "instrument handle"=w608) -> ()  [unwired: 7 in, 2 out]
          }
        }
        n310 = case shown="False" w592 {
          tunnel: w594 -> [_ w620]
          frame False {
          }
          frame True {
            n311 = call <instrlib>:"niDCPower Configure Output Enabled.vi"("output enabled"=TRUE ("V0.0"), "channel name"="1", "instrument handle"=w620) -> ()  [unwired: 7 in, 2 out]
          }
        }
        n312 = case shown="False" w589 {
          tunnel: w580 -> [_ w614]
          frame False {
          }
          frame True {
            n313 = call <instrlib>:"niDCPower Configure Output Enabled.vi"("output enabled"=TRUE ("V0.0"), "channel name"="0", "instrument handle"=w614) -> ()  [unwired: 7 in, 2 out]
          }
        }
        n314 = case shown="False" w604 {
          frame False {
          }
          frame True {
            w630 = TRUE
            n315 = local write "V1.0"(w630) -> ()
            n316 = local write "V1.1"(w630) -> ()
            n317 = local write "V0.1"(w630) -> ()
            n318 = local write "V0.0"(w630) -> ()
          }
        }
        n319 = case shown="False" w603 {
          frame False {
          }
          frame True {
            w629 = FALSE
            n320 = local write "V1.0"(w629) -> ()
            n321 = local write "V1.1"(w629) -> ()
            n322 = local write "V0.1"(w629) -> ()
            n323 = local write "V0.0"(w629) -> ()
          }
        }
        n324 = case shown="False" w595 {
          tunnel: w594 -> [_ w623]
          frame False {
          }
          frame True {
            n325 = call <instrlib>:"niDCPower Configure Output Enabled.vi"("output enabled"=FALSE ("V0.0"), "channel name"="0", "instrument handle"=w623) -> ()  [unwired: 7 in, 2 out]
          }
        }
        n326 = case shown="False" w581 {
          tunnel: w580 -> [_ w605]
          frame False {
          }
          frame True {
            n327 = call <instrlib>:"niDCPower Configure Output Enabled.vi"("output enabled"=FALSE ("V0.0"), "channel name"="1", "instrument handle"=w605) -> ()  [unwired: 7 in, 2 out]
          }
        }
        n328 = case shown="False" w591 {
          tunnel: w594 -> [_ w617]
          frame False {
          }
          frame True {
            n329 = call <instrlib>:"niDCPower Configure Output Enabled.vi"("output enabled"=FALSE ("V0.0"), "channel name"="1", "instrument handle"=w617) -> ()  [unwired: 7 in, 2 out]
          }
        }
        n330 = case shown="False" w588 {
          tunnel: w580 -> [_ w611]
          frame False {
          }
          frame True {
            n331 = call <instrlib>:"niDCPower Configure Output Enabled.vi"("output enabled"=FALSE ("V0.0"), "channel name"="0", "instrument handle"=w611) -> ()  [unwired: 7 in, 2 out]
          }
        }
      }
      frame #2 {
      }
    }
    n332 = Wait (ms)(milliseconds to wait=u32 1) -> ()  [unwired: 1 out]
  }
  n333 = flat-sequence {
    tunnel: w12 -> [w634]
    tunnel: w11 -> [w649]
    tunnel: w13 -> [w635]
    tunnel: w8 -> [w636]
    tunnel: w7 -> [w637]
    tunnel: w6 -> [w638]
    tunnel: w5 -> [w633]
    frame #0 {
      # "Завершение работы программы"
      n334 = Close File(refnum=w633) -> ()  [unwired: 1 in, 2 out]
      n335 = Unregister For Events(event registration refnum=w634) -> (error out=w656:errorcluster)  [unwired: 1 in]
      n336 = local write "CheckSeeDone"(TRUE ("StartCheckSee")) -> ()
      n337 = local write "ExamineSeeDone"(TRUE ("StartCheckSee")) -> ()
      n338 = local write "ShutdownDone"(TRUE ("StartCheckSee")) -> ()
      n339 = local write "TryParrySeeDone"(TRUE ("StartCheckSee")) -> ()
      n340 = invoke class="RemoteSeeAbleService" method="Dispose"(reference=w649, error in=w656) -> (reference out=w655:refnum<k24>, error out=w654:errorcluster)  [unwired: 1 in, 1 out]
      n341 = call <instrlib>:"niDCPower Abort.vi"("error in (no error)"=w637, "instrument handle"=w638) -> ("error out"=w639:errorcluster, "instrument handle out"=w640:refnum<k15>)  [unwired: 8 in]
      n342 = call <instrlib>:"niDCPower Abort.vi"("error in (no error)"=w635, "instrument handle"=w636) -> ("error out"=w642:errorcluster, "instrument handle out"=w641:refnum<k15>)  [unwired: 8 in]
      n343 = call <instrlib>:"niDCPower Reset Device.vi"("error in (no error)"=w642, "instrument handle"=w641) -> ("error out"=w646:errorcluster, "instrument handle out"=w647:refnum<k15>)  [unwired: 8 in]
      n344 = call <instrlib>:"niDCPower Reset Device.vi"("error in (no error)"=w639, "instrument handle"=w640) -> ("error out"=w645:errorcluster, "instrument handle out"=w644:refnum<k15>)  [unwired: 8 in]
      n345 = call <instrlib>:"niDCPower Close.vi"("error in (no error)"=w646, "instrument handle"=w647) -> ("error out"=w648:errorcluster)  [unwired: 9 in]
      n346 = call <instrlib>:"niDCPower Close.vi"("error in (no error)"=w645, "instrument handle"=w644) -> ("error out"=w643:errorcluster)  [unwired: 9 in]
      n347 = call <vilib>:"Simple Error Handler.vi"("error in (no error)"=w648) -> ()  [unwired: 1 in, 8 out]
      n348 = call <vilib>:"Simple Error Handler.vi"("error in (no error)"=w643) -> ()  [unwired: 1 in, 8 out]
      n349 = Close Reference(reference=w655, error in (no error)=w654) -> ()  [unwired: 1 out]
    }
  }
